vi "test Fails If Months Are Not Equal.vi"(8 "error in (no error)":errorcluster, 11 "TestCase in":refnum<class "Timestamp Comparison Test Case.lvclass">) -> (0 "error out":errorcluster, 3 "TestCase out":refnum<class "Timestamp Comparison Test Case.lvclass">)   [LabVIEW 2015, in "Timestamp Comparison Test Case.lvclass"]
uses:
  Timestamp Comparison Test Case.lvclass
  <vilib>/addons/_JKI Toolkits/VI Tester/TestCase.llb/TestCase.lvclass
  VITAC.lvlib
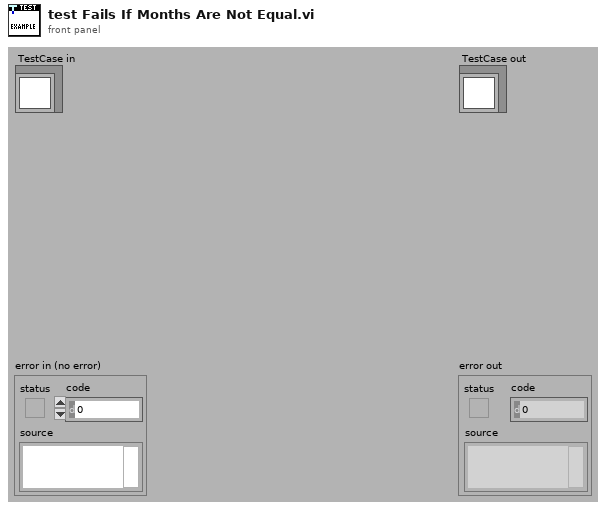
[diagram p1: front panel]
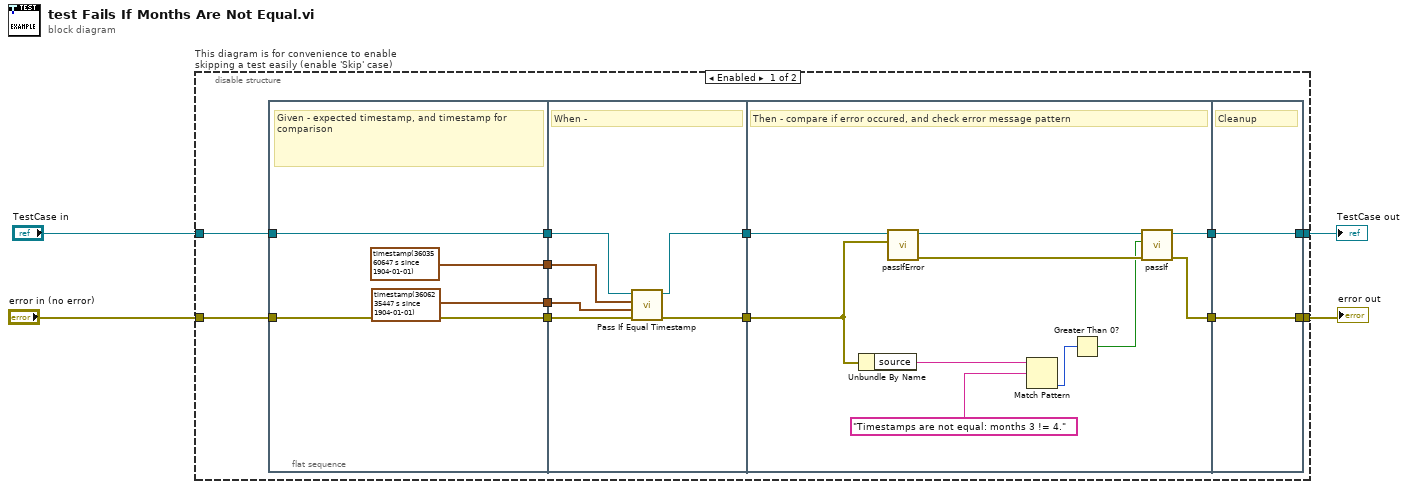
[diagram p0: block diagram]
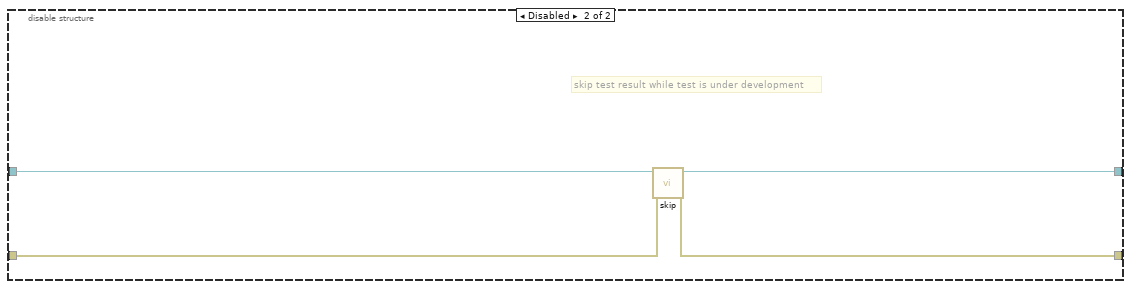
[diagram p2: hidden frame]
diagram:
  n1 = disable-structure "This diagram is for convenience to enable skipping a test easily (enable 'Skip' case)" shown="Enabled" {
    disable-tunnel: "TestCase in" -> [w8 w42]
    disable-tunnel: [w10 w40] -> w1
    disable-tunnel: [w9 w41] -> w3
    disable-tunnel: "error in (no error)" -> [w7 w39]
    frame Enabled {
      n2 = flat-sequence {
        tunnel: w7 -> [w19]
        tunnel: w8 -> [w20]
        tunnel: [w20] -> w16
        tunnel: [w19] -> w15
        tunnel: [timestamp(3603560647.1 s since 1904-01-01) ("current time")] -> w6
        tunnel: [timestamp(3606235447.1 s since 1904-01-01) ("current time")] -> w5
        tunnel: [w23] -> w14
        tunnel: [w25] -> w13
        tunnel: w16 -> [w24]
        tunnel: w15 -> [w26]
        tunnel: w6 -> [w22]
        tunnel: w5 -> [w21]
        tunnel: [w27] -> w12
        tunnel: w14 -> [w30]
        tunnel: w13 -> [w29]
        tunnel: [w28] -> w11
        tunnel: [w37] -> w9
        tunnel: [w38] -> w10
        tunnel: w12 -> [w38]
        tunnel: w11 -> [w37]
        frame #0 {
          # "Given - expected timestamp, and timestamp for comparison"
        }
        frame #1 {
          # "When -"
          n3 = call "Pass If Equal Timestamp.vi"("error in (no error)"=w26, "actual timestamp"=w21, "expected timestamp"=w22, "TestCase in"=w24) -> ("error out"=w25:errorcluster, "TestCase out"=w23:refnum<class "Timestamp Comparison Test Case.lvclass">)  [unwired: 6 in]
        }
        frame #2 {
          # "Then - compare if error occured, and check error message pattern"
          n4 = Unbundle By Name(w29) -> ("source"=w34:string)
          n5 = call-dynamic "passIfError.vi"("error"=w29, "TestCase in"=w30) -> ("error out"=w35:errorcluster, "TestCase out"=w36:refnum<class "Timestamp Comparison Test Case.lvclass">)  [unwired: 8 in]
          n6 = Match Pattern(string=w34, regular expression="Timestamps are not equal: months 3 != 4.") -> (offset past match=w32:i32)  [unwired: 1 in, 3 out]
          n7 = Greater Than 0?(x=w32) -> (x > 0?=w31:bool)
          n8 = call-dynamic "passIf.vi"("error in (no error)"=w35, "pass"=w31, "TestCase in"=w36) -> ("error out"=w28:errorcluster, "TestCase out"=w27:refnum<class "Timestamp Comparison Test Case.lvclass">)  [unwired: 7 in]
        }
        frame #3 {
          # "Cleanup"
        }
      }
    }
    frame Disabled {
      # "skip test result while test is under development"
      n9 = call <vilib>:"skip.vi"("error in (no error)"=w39, "TestCase in"=w42) -> ("error out"=w41:errorcluster, "TestCase out"=w40:refnum<class "Timestamp Comparison Test Case.lvclass">)  [unwired: 8 in]
    }
  }
  "error out" <- w3
  "TestCase out" <- w1
